vi "Get XML (Prettyprint).vi"(8 "error in (no error)":errorcluster, 11 "DOM document in":refnum<k20>) -> (0 "error out":errorcluster, 2 "pretty formatted XML":string, 3 "DOM document out":refnum<k20>)   [LabVIEW 2017, in "Error File Management.lvlib"]
uses:
  Error File Management.lvlib
  <resource>/objmgr/DOMUserDefRef.rc
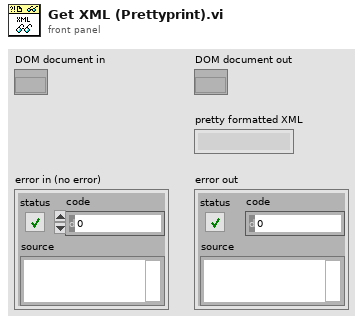
[diagram p1: front panel]
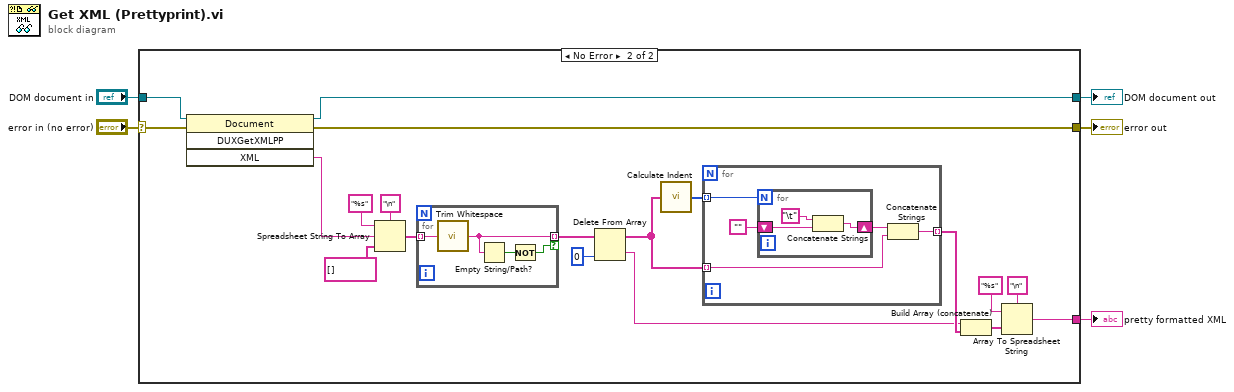
[diagram p0: block diagram]
diagram:
  n1 = case shown="No Error" "error in (no error)" {
    selector: "error in (no error)" -> [w7 w10]
    tunnel: [_ w20] -> w5
    tunnel: [w7 w11] -> w3
    tunnel: "DOM document in" -> [w6 w9]
    tunnel: [w6 w8] -> w1
    frame Error {
    }
    frame No Error {
      n2 = invoke class="Document" method="DUXGetXMLPP"(reference=w9, error in=w10) -> (reference out=w8:refnum<k20>, error out=w11:errorcluster, "XML"=w17:string)  [unwired: 2 in, 1 out]
      n3 = Spreadsheet String To Array(delimiter (Tab)="\n", format string="%s", spreadsheet string=w17, array type (2D Dbl)=string[] []) -> (array=w13:string[])
      n4 = for {
        tunnel: w13 -> [w30] mode=indexing
        tunnel: [w29] -> w12 mode=indexing if=w27
        n5 = call <vilib>:"Trim Whitespace.vi"("string"=w30) -> ("trimmed string"=w29:string)  [unwired: 1 in]
        n6 = Empty String/Path?(string/path=w29) -> (empty?=w28:bool)
        n7 = Not(x=w28) -> (.not. x?=w27:bool)
      }
      n8 = Delete From Array(array=w12, index=0) -> (deleted portion=w18:string, array with subset deleted=w24:string[])  [unwired: 1 in]
      n9 = call "Calculate Indent.vi"("input"=w24) -> ("indent"=w25:i32[])
      n10 = for {
        tunnel: w25 -> [w35] mode=indexing
        tunnel: w24 -> [w32] mode=indexing
        tunnel: [w31] -> w23 mode=indexing
        n11 = for {
          N: w35 -> [_]
          shift-right: [w37] -> w33
          shift-left: "" -> [w36]
          n12 = Concatenate Strings("\t", w36) -> (w37:string)
        }
        n13 = Concatenate Strings(w33, w32) -> (w31:string)
      }
      n14 = Build Array (concatenate)(w18, w23) -> (w19:string[])
      n15 = Array To Spreadsheet String(delimiter (Tab)="\n", array=w19, 3:"%s" ("format string")) -> (spreadsheet string=w20:string)
    }
  }
  "pretty formatted XML" <- w5
  "error out" <- w3
  "DOM document out" <- w1
